vi "U16 Two's Compliment To Decimal.vi"(3 "Two's Compliment U16":u16) -> (1 "Decimal I16":i16)   [LabVIEW 2011, in "LMH-Toolbox.lvlib" / "LMH-Common.lvlib"]
doc: "Convert a U16 in Two's compliment into a decimal number."
uses:
  LMH-Common.lvlib
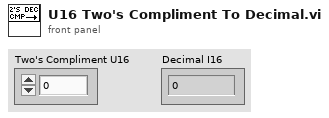
[diagram p1: front panel]
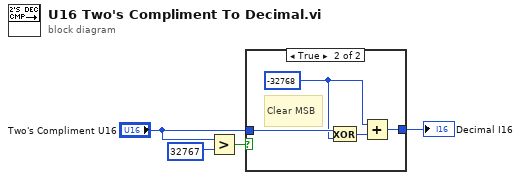
[diagram p0: block diagram]
diagram:
  n1 = Greater?(x="Two's Compliment U16", y=u16 32767) -> (0:w3:bool)
  n2 = case shown="True" w3 {
    tunnel: "Two's Compliment U16" -> [w5 w8]
    tunnel: [w5 w9] -> w2
    frame False {
    }
    frame True {
      w6 = i16 -32768 ("y")
      # "Clear MSB"
      n3 = Exclusive Or(1:w6, 2:w8) -> (0:w7:u16)
      n4 = Add(x=w6, y=w7) -> (x+y=w9:u16)
    }
  }
  "Decimal I16" <- w2
